vi "Stop Core.vi"(10 "final error code":i32, 11 "CO2 Actor in":refnum<class "CO2 Actor.lvclass">) -> (3 "CO2 Actor out":refnum<class "CO2 Actor.lvclass">)   [LabVIEW 2015, in "cRIO-Carbondioxide.lvlib" / "CO2-Actor.lvlib" / "CO2 Actor.lvclass"]
doc: "(<B>Filename</B>: Actor Framework.lvlib:Actor.lvclass:Stop Core.vi)\n\nDefines what the actor does before it stops. Use the <B>final error code</B> input to determine whether the actor shut down in response to an error.\n\nBy default, this method does nothing. A descendant class may override it to define behavior, such as shutting down any processes the actor initiated in its override of the Actor Core method."
uses:
  CO2 Actor.lvclass
  CO2 Actor.lvclass/CO2 Actor.ctl
  <vilib>/ActorFramework/Actor/Actor.lvclass
  cRIO-CO2 Messages/Unregister Actor Msg/Unregister Actor Msg.lvclass
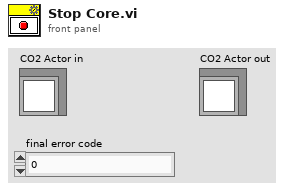
[diagram p1: front panel]
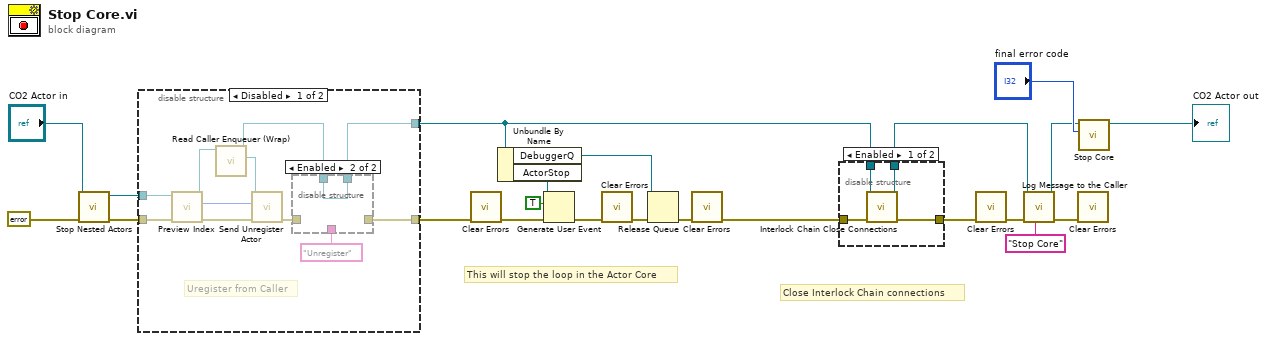
[diagram p0: block diagram]
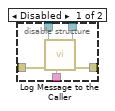
[diagram p2: hidden frame]
diagram:
  # "Close Interlock Chain connections"
  # "This will stop the loop in the Actor Core"
  n1 = call-dynamic "Stop Nested Actors.vi"("error in (no error)"=errorcluster {"status"=FALSE, "code"=0, "source"=""}, "CO2 Actor in"="CO2 Actor in") -> ("error out"=w6:errorcluster, "CO2 Actor out"=w4:refnum<class "CO2 Actor.lvclass">)  [unwired: 8 in]
  n2 = disable-structure shown="Disabled" {
    disable-tunnel: [w27 w40] -> w13
    disable-tunnel: [w25 w41] -> w3
    disable-tunnel: w6 -> [w24 w40]
    disable-tunnel: w4 -> [w23 w41]
    frame Disabled {
      # "Uregister from Caller"
      n3 = call "Preview Index.vi"("error in (no error)"=w24, "CO2 Actor in"=w23) -> ("error out"=w32:errorcluster, "Index"=w31:i32, "CO2 Actor out"=w29:refnum<class "CO2 Actor.lvclass">)  [unwired: 7 in]
      n4 = call "Read Caller Enqueuer (Wrap).vi"("CO2 Actor in"=w29) -> ("Actor Framework:Message Enqueuer"=w33:refnum<class "Message Enqueuer.lvclass">, "CO2 Actor out"=w26:refnum<class "CO2 Actor.lvclass">)  [unwired: 9 in]
      n5 = call "Send Unregister Actor.vi"("error in (no error)"=w32, "Index"=w31, "Message Enqueuer"=w33) -> ("error out"=w28:errorcluster)  [unwired: 7 in, 1 out]
      n6 = disable-structure shown="Enabled" {
        disable-tunnel: "Unregister" ("String (\"OK\")") -> [w38 _]
        disable-tunnel: w28 -> [w37 _]
        disable-tunnel: [w36 _] -> w27
        disable-tunnel: w26 -> [w35 w39]
        disable-tunnel: [w34 w39] -> w25
        frame Disabled {
          n7 = call-dynamic "Log Message to the Caller.vi"("String (\"\" = no message to send)"=w38, "error in (no error)"=w37, "CO2 Actor in"=w35) -> ("error out"=w36:errorcluster, "CO2 Actor out"=w34:refnum<class "CO2 Actor.lvclass">)  [unwired: 7 in]
        }
        frame Enabled {
        }
      }
    }
    frame Enabled {
    }
  }
  n8 = call <vilib>:"Clear Errors.vi"("error in (no error)"=w13) -> ("error out"=w12:errorcluster)  [unwired: 5 in, 1 out]
  n9 = Unbundle By Name(w3) -> ("DebuggerQ"=w18:refnum<queue>, "ActorStop"=w21:refnum<user-event>)
  n10 = Generate User Event(user event=w21, event data cluster=TRUE ("event data"), error in=w12) -> (error out=w20:errorcluster)  [unwired: 1 in, 1 out]
  n11 = call <vilib>:"Clear Errors.vi"("error in (no error)"=w20) -> ("error out"=w19:errorcluster)  [unwired: 5 in, 1 out]
  n12 = Release Queue(queue=w18, error in (no error)=w19) -> (error out=w17:errorcluster)  [unwired: 1 in, 2 out]
  n13 = call <vilib>:"Clear Errors.vi"("error in (no error)"=w17) -> ("error out"=w2:errorcluster)  [unwired: 5 in, 1 out]
  n14 = disable-structure shown="Enabled" {
    disable-tunnel: w2 -> [w45 _]
    disable-tunnel: [w44 _] -> w11
    disable-tunnel: w3 -> [w43 w46]
    disable-tunnel: [w42 w46] -> w10
    frame Enabled {
      n15 = call "Interlock Chain Close Connections.vi"("error in (no error)"=w45, "CO2 Actor in"=w43) -> ("error out"=w44:errorcluster, "CO2 Actor out"=w42:refnum<class "CO2 Actor.lvclass">)  [unwired: 8 in]
    }
    frame Disabled {
    }
  }
  n16 = call <vilib>:"Clear Errors.vi"("error in (no error)"=w11) -> ("error out"=w9:errorcluster)  [unwired: 5 in, 1 out]
  n17 = call-dynamic "Log Message to the Caller.vi"("String (\"\" = no message to send)"="Stop Core" ("String (\"OK\")"), "error in (no error)"=w9, "CO2 Actor in"=w10) -> ("error out"=w8:errorcluster, "CO2 Actor out"=w14:refnum<class "CO2 Actor.lvclass">)  [unwired: 7 in]
  n18 = call <vilib>:"Clear Errors.vi"("error in (no error)"=w8) -> ()  [unwired: 5 in, 2 out]
  n19 = call-parent "Stop Core.vi"("final error code"="final error code", "Actor in"=w14) -> ("Actor out"=→"CO2 Actor out":refnum<class "CO2 Actor.lvclass">)  [unwired: 9 in]
